vi "Test Histogram.vi"(6 "Obsticle Clearence":dbl, 8 "Threshold":dbl, 9 "Desired Heading (degrees)":dbl, 10 "Magnitude In (m)":dbl[](array[numeric]), 11 "Angles In (degrees)":dbl[](array[numeric])) -> (0 "Mask out":bool[](array[boolean]), 3 "Command Heading":dbl)   [LabVIEW 2011]
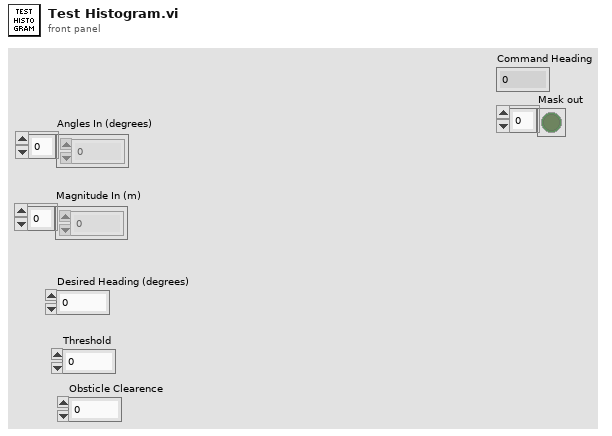
[diagram p1: front panel]
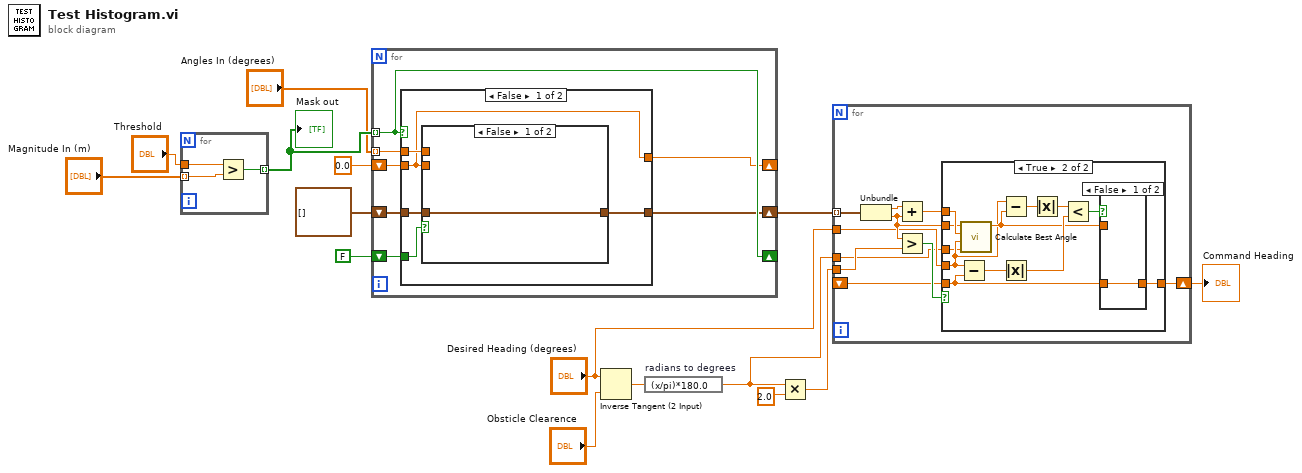
[diagram p0: block diagram]
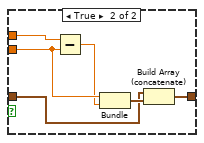
[diagram p4: hidden frame]
diagram:
  n1 = for {
    tunnel: "Magnitude In (m)" -> [w18] mode=indexing
    tunnel: "Threshold" -> [w17]
    tunnel: [w16] -> w11 mode=indexing
    n2 = Greater?(x=w17, y=w18) -> (0:w16:bool)
  }
  "Mask out" <- w11
  n3 = for {
    tunnel: w11 -> [w25] mode=indexing
    tunnel: "Angles In (degrees)" -> [w23] mode=indexing
    shift-right: [w25] -> _
    shift-left: FALSE -> [w24]
    shift-right: [w22] -> _
    shift-left: 0.0 ("Numeric") -> [w21]
    shift-right: [w20] -> w6
    shift-left: cluster{"Numeric":dbl, dbl}[] [] -> [w19]
    n4 = case shown="False" w25 {
      tunnel: w24 -> [w30 w42]
      tunnel: w23 -> [w28 w41]
      tunnel: [w26 w40] -> w22
      tunnel: w21 -> [w26 w39]
      tunnel: [w29 w38] -> w20
      tunnel: w19 -> [w27 w38]
      frame False {
        n5 = case shown="False" w30 {
          tunnel: [w31 w37] -> w29
          tunnel: w26 -> [_ w35]
          tunnel: w28 -> [_ w34]
          tunnel: w27 -> [w31 w32]
          frame False {
          }
          frame True {
            n6 = Subtract(x=w34, y=w35) -> (x-y=w33:dbl)
            n7 = Bundle("Numeric"=w35, w33) -> (w36:cluster{"Numeric":dbl, dbl})  [unwired: 1 in]
            n8 = Build Array (concatenate)(w32, w36) -> (w37:cluster{"Numeric":dbl, dbl}[])
          }
        }
      }
      frame True {
        n9 = case shown="True" w42 {
          tunnel: w41 -> [w43 _]
          tunnel: [w43 w44] -> w40
          tunnel: w39 -> [_ w44]
          frame False {
          }
          frame True {
          }
        }
      }
    }
  }
  n10 = Inverse Tangent (2 Input)(1:"Obsticle Clearence", 2:"Desired Heading (degrees)") -> (0:w12:dbl)
  n11 = expression code="(x/pi)*180.0" "radians to degrees"(w12) -> (w1:dbl)
  n12 = Multiply(x=w1, y=2.0) -> (x*y=w4:dbl)
  n13 = for {
    tunnel: w6 -> [w54] mode=indexing
    tunnel: w4 -> [w53]
    shift-right: [w46] -> w3
    shift-left: _ -> [w47]
    tunnel: "Desired Heading (degrees)" -> [w48]
    tunnel: w1 -> [w45]
    n14 = Unbundle(w54) -> ("Numeric"=w51:dbl, w49:dbl)
    n15 = Add(x=w51, y=w49) -> (x+y=w50:dbl)
    n16 = Greater?(x=w49, y=w53) -> (0:w52:bool)
    n17 = case shown="True" w52 {
      tunnel: w50 -> [_ w67]
      tunnel: w49 -> [_ w66]
      tunnel: w48 -> [_ w57]
      tunnel: w47 -> [w55 w58]
      tunnel: [w55 w60] -> w46
      tunnel: w45 -> [_ w56]
      frame False {
      }
      frame True {
        n18 = Subtract(x=w57, y=w58) -> (x-y=w64:dbl)
        n19 = call "Calculate Best Angle.vi"("Bearing Clearence"=w56, "Desired Bearing"=w57, "Angle (max)"=w67, "Angle (min)"=w66) -> ("Command Heading"=w59:dbl)  [unwired: 7 in]
        n20 = Subtract(x=w57, y=w59) -> (x-y=w65:dbl)
        n21 = Absolute Value(x=w64) -> (abs(x)=w63:dbl)
        n22 = Absolute Value(x=w65) -> (abs(x)=w62:dbl)
        n23 = Less?(x=w62, y=w63) -> (x < y?=w61:bool)
        n24 = case shown="False" w61 {
          tunnel: [w68 w69] -> w60
          tunnel: w59 -> [_ w69]
          tunnel: w58 -> [w68 _]
          frame False {
          }
          frame True {
          }
        }
      }
    }
  }
  "Command Heading" <- w3
